vi "palindrome labview.vi"() -> ()   [LabVIEW 2015]
panel:
  out "IS A PALINDROME OR NOT":string
  out "REVERSE STRING":string
  in  "String":string
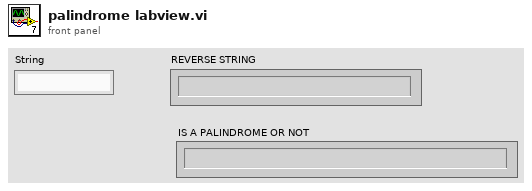
[diagram p1: front panel]
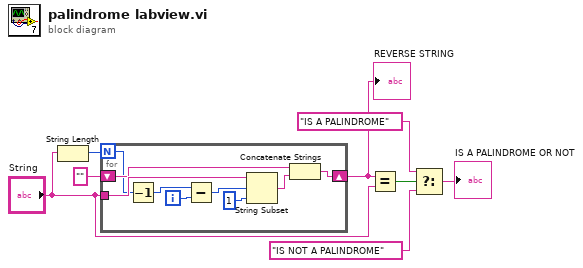
[diagram p0: block diagram]
diagram:
  n1 = String Length(string="String") -> (length=w8:i32)
  n2 = for {
    N: w8 -> [w10]
    tunnel: "String" -> [w16]
    shift-right: [w12] -> w6
    shift-left: "" -> [w11]
    i -> [w17]
    n3 = Decrement(x=w10) -> (x-1=w9:i32)
    n4 = Subtract(x=w9, y=w17) -> (x-y=w14:i32)
    n5 = String Subset(string=w16, offset (0)=w14, length (rest)=1 ("length (rest)")) -> (substring=w13:string)
    n6 = Concatenate Strings(w11, w13) -> (w12:string)
  }
  "REVERSE STRING" <- w6
  n7 = Equal?(x=w6, y="String") -> (x = y?=w4:bool)
  n8 = Select(t="IS A PALINDROME", s=w4, f="IS NOT A PALINDROME") -> (s? t:f=→"IS A PALINDROME OR NOT":string)
